vi "配置信息读取.vi"(8 "error in (no error)":errorcluster caption="错误输入（无错误）") -> (0 "error out":errorcluster caption="错误输出")   [LabVIEW 2016, in "质控单元V4.lvlib"]
uses:
  <vilib>/Utility/config.llb/NI_LVConfig.lvlib
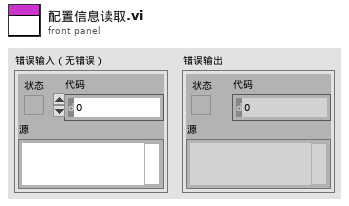
[diagram p1: front panel]
types:
  T1 = typedef "NI_LVConfig.lvlib/Config Data RefNum.ctl" = refnum<k1>
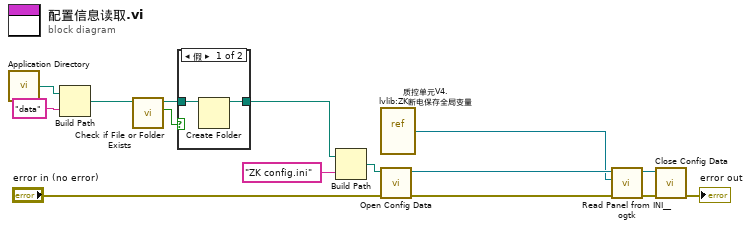
[diagram p0: block diagram]
diagram:
  n1 = call <vilib>:"Application Directory.vi"() -> ("Application Directory"=w12:path)
  n2 = Build Path(base path=w12, name or relative path="data" ("名称或相对路径")) -> (appended path=w10:path)
  n3 = call <vilib>:"Check if File or Folder Exists.vi"("path"=w10) -> ("file or folder exists?"=w9:bool, "dup path"=w8:path)  [unwired: 8 in, 1 out]
  n4 = case shown="假" w9 {
    tunnel: w8 -> [w17 w18]
    tunnel: [w16 w18] -> w7
    frame False {
      n5 = Create Folder(path (use dialog)=w17) -> (created path=w16:path)  [unwired: 2 in, 2 out]
    }
    frame True {
    }
  }
  n6 = Build Path(base path=w7, name or relative path="ZK config.ini" ("名称或相对路径")) -> (appended path=w5:path)
  n7 = vi-ref "质控单元V4.lvlib:ZK断电保存全局变量.vi"() -> (w13:refnum<vi>)
  n8 = call <vilib>:"Open Config Data.vi"("error in (no error)"="error in (no error)", "configuration file path"=w5) -> ("error out"=w15:errorcluster, "refnum"=w14:T1)  [unwired: 7 in, 1 out]
  n9 = call <userlib>:"Read Panel from INI__ogtk.vi"("error in (no error)"=w15, "VI ref"=w13, "refnum"=w14) -> ("error out"=w4:errorcluster, "refnum out"=w3:T1)  [unwired: 7 in]
  n10 = call <vilib>:"Close Config Data.vi"("error in (no error)"=w4, "refnum"=w3) -> ("error out"=→"error out":errorcluster)  [unwired: 8 in, 1 out]
